vi "Read.vi"(0 "RBD9103":T3, 5 "error in":errorcluster) -> (11 "Command time, ms":u32, 14 "RBD9103 out":T3, 15 "Quality":T2, 16 "Range out":T1 items=["Auto range", "2nA", "20nA", "200nA", "2uA", "20uA", "200uA", "2mA"], 17 "Value, nA":dbl, 19 "error out":errorcluster)   [LabVIEW 2018]
uses:
  RBD9103.ctl
  GenericDataEvent/GenericEvent.ctl
  Quality.ctl
  Range.ctl
  Operation type.ctl
panel:
  out "Time, mc":u32
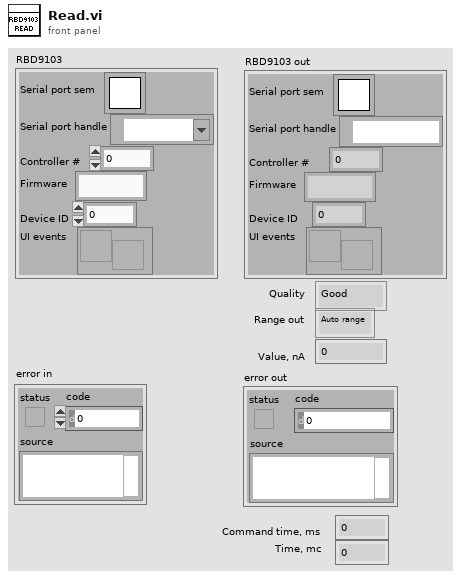
[diagram p1: front panel]
types:
  T1 = typedef "Range.ctl" = u16
  T2 = typedef "Quality.ctl" = enum16{"Good", "Unstable", "Under", "Over"}
  T3 = typedef "RBD9103.ctl" = cluster{"Serial port sem":T4, "Serial port handle":refnum<visa-resource-name>, "Controller #":u8, "Firmware":string, "Device ID":i32, "UI events":T5}
  T4 = typedef "Semaphore RefNum" = refnum<k1>
  T5 = typedef "GenericEvent.ctl" = refnum<user-event>
  T6 = typedef "Operation type.ctl" = enum16{"Write&Read", "Read only", "Write only", "Read only multiply"}
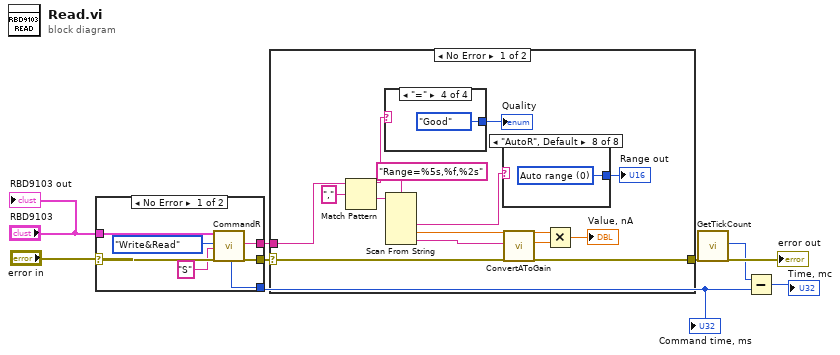
[diagram p0: block diagram]
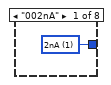
[diagram p2: hidden frame]
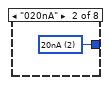
[diagram p3: hidden frame]
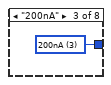
[diagram p4: hidden frame]
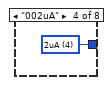
[diagram p5: hidden frame]
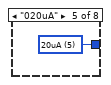
[diagram p6: hidden frame]
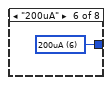
[diagram p7: hidden frame]
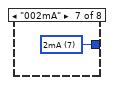
[diagram p8: hidden frame]
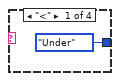
[diagram p9: hidden frame]
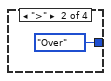
[diagram p10: hidden frame]
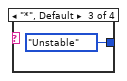
[diagram p11: hidden frame]
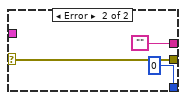
[diagram p13: hidden frame]
diagram:
  n1 = case shown="No Error" "error in" {
    selector: "error in" -> [w15 w19]
    tunnel: [w14 w19] -> w7
    tunnel: "RBD9103" -> [w16 _]
    tunnel: [w11 ""] -> w6
    tunnel: [w10 u32 0 ("Command time, ms")] -> w2
    frame No Error {
      n2 = call "CommandR.vi"("RBD9103"=w16, "Operation"=Operation_type."Write&Read" ("Operation type"), "Command"="S", "error in"=w15) -> ("Command time, ms"=w10:u32, "Answer"=w11:string, "error out"=w14:errorcluster)  [unwired: 12 in, 1 out]
    }
    frame Error {
    }
  }
  "Command time, ms" <- w2
  n3 = case shown="No Error" w7 {
    selector: w7 -> [w24 w46]
    tunnel: [w28 w46] -> w5
    tunnel: w6 -> [w31 _]
    frame No Error {
      n4 = Match Pattern(string=w31, regular expression=",") -> (before substring=w30:string, after substring=w32:string)  [unwired: 1 in, 2 out]
      n5 = case shown="\"=\"" w30 {
        tunnel: [Quality."Under" ("Quality") Quality."Over" ("Quality") Quality."Unstable" ("Quality") Quality."Good" ("Quality")] -> w29
        frame "<" {
        }
        frame ">" {
        }
        frame "*", Default {
        }
        frame "=" {
        }
      }
      "Quality" <- w29
      n6 = Scan From String(format string="Range=%5s,%f,%2s", input string=w32) -> (output 1=w21:string, output 2=w23:dbl, output 3=w22:string)  [unwired: 5 in, 3 out]
      n7 = case shown="\"AutoR\", Default" w21 {
        tunnel: [w34 w35 w36 w37 w38 w39 w40 w41] -> w20
        frame "002nA" {
          w34 = T1 1 items=["Auto range", "2nA", "20nA", "200nA", "2uA", "20uA", "200uA", "2mA"] ("Range out")
        }
        frame "020nA" {
          w35 = T1 2 items=["Auto range", "2nA", "20nA", "200nA", "2uA", "20uA", "200uA", "2mA"] ("Range out")
        }
        frame "200nA" {
          w36 = T1 3 items=["Auto range", "2nA", "20nA", "200nA", "2uA", "20uA", "200uA", "2mA"] ("Range out")
        }
        frame "002uA" {
          w37 = T1 4 items=["Auto range", "2nA", "20nA", "200nA", "2uA", "20uA", "200uA", "2mA"] ("Range out")
        }
        frame "020uA" {
          w38 = T1 5 items=["Auto range", "2nA", "20nA", "200nA", "2uA", "20uA", "200uA", "2mA"] ("Range out")
        }
        frame "200uA" {
          w39 = T1 6 items=["Auto range", "2nA", "20nA", "200nA", "2uA", "20uA", "200uA", "2mA"] ("Range out")
        }
        frame "002mA" {
          w40 = T1 7 items=["Auto range", "2nA", "20nA", "200nA", "2uA", "20uA", "200uA", "2mA"] ("Range out")
        }
        frame "AutoR", Default {
          w41 = T1 0 items=["Auto range", "2nA", "20nA", "200nA", "2uA", "20uA", "200uA", "2mA"] ("Range out")
        }
      }
      "Range out" <- w20
      n8 = call "ConvertAToGain.vi"("String"=w22, "error in"=w24) -> ("Gain"=w27:dbl, "error out"=w28:errorcluster)  [unwired: 16 in]
      n9 = Multiply(x=w23, y=w27) -> (x*y=→"Value, nA":dbl)
    }
    frame Error {
    }
  }
  n10 = call "GetTickCount.vi"("error in (no error)"=w5) -> ("ms"=w3:u32, "error IO"=→"error out":errorcluster)  [unwired: 17 in]
  n11 = Subtract(x=w3, y=w2) -> (x-y=→"Time, mc":u32)
  "RBD9103 out" <- "RBD9103"
